vi "Train.vi"(6 "Parallel Instances (8)":i32=8, 7 "Queue in":refnum<queue>, 8 "error in (no error)":errorcluster, 9 "Progress ref in":refnum<vi>, 10 "File Data Array":T1[](array[typedef]), 11 "MarkovModel in":refnum<class "MarkovModel.lvclass">) -> (0 "error out":errorcluster, 3 "MarkovModel out":refnum<class "MarkovModel.lvclass">)   [LabVIEW 2020, in "MarkovModel.lvclass"]
uses:
  MarkovModel.lvclass
  MarkovModel.lvclass/MarkovModel.ctl
  File Metadata.ctl
  Node.ctl
  Source to Sink Array.ctl
  File Data.ctl
  Indexer Action.ctl
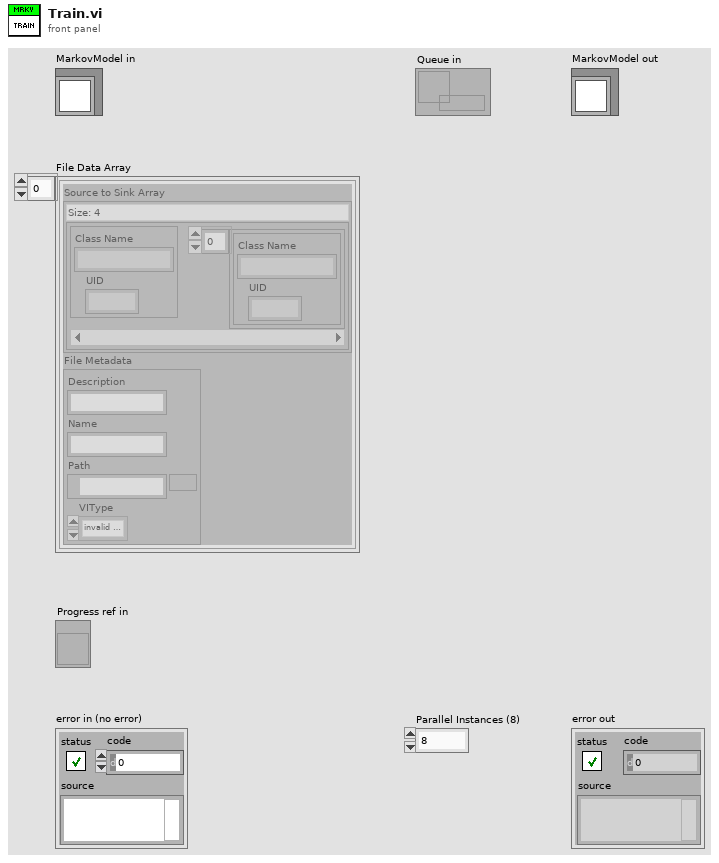
[diagram p1: front panel]
types:
  T1 = typedef "File Data.ctl" = cluster{"Source to Sink Array":T2, "File Metadata":T4}
  T2 = typedef "Source to Sink Array.ctl" = map{T3, T3[]}
  T3 = typedef "Node.ctl" = cluster{"Class Name":string, "UID":i32}
  T4 = typedef "File Metadata.ctl" = cluster{"Description":string, "Name":string, "Path":path, "VIType":enum32{"invalid VI type", "Standard VI", "Control VI", "Global VI", "Polymorphic VI", "Configuration VI", "SubSystem", "Facade VI", "Method VI", "Statechart Diagram VI"}}
  T5 = map{string[], cluster{"Class Name":string, "Count":i32}[]}
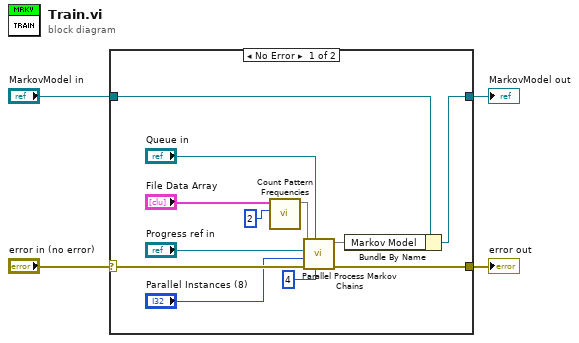
[diagram p0: block diagram]
diagram:
  n1 = case shown="No Error" "error in (no error)" {
    selector: "error in (no error)" -> [w11 w18]
    tunnel: [w14 w18] -> w3
    tunnel: "MarkovModel in" -> [w16 w17]
    tunnel: [w15 w17] -> w1
    frame No Error {
      n2 = call "Count Pattern Frequencies.vi"("Order"=2, "File Data Array"="File Data Array") -> ("Pattern Frequencies"=w12:map{string[], i32})  [unwired: 9 in]
      n3 = call "Parallel Process Markov Chains.vi"("Suggestion Limit"=u16 4, "Queue in"="Queue in", "error in (no error)"=w11, "Parallel Instances (8)"="Parallel Instances (8)", "Progress ref in"="Progress ref in", "Pattern Frequencies"=w12) -> ("error out"=w14:errorcluster, "Map"=w13:T5)  [unwired: 4 in]
      n4 = Bundle By Name(cluster=w16, "Markov Model"=w13) -> (w15:refnum<class "MarkovModel.lvclass">)
    }
    frame Error {
    }
  }
  "error out" <- w3
  "MarkovModel out" <- w1
